vi "PRY_to_Quat.vi"(1 "From Degrees? (T)":bool=TRUE, 2 "Orientation":T1) -> (0 "Quaternion":cluster{"x":dbl, "y":dbl, "z":dbl, "w":dbl})   [LabVIEW 2014]
doc: "Converts a Pitch, Roll, Yaw orientation to a Quaternion"
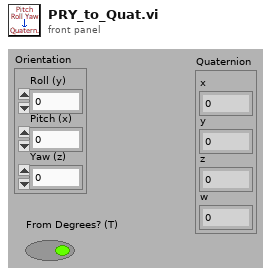
[diagram p1: front panel]
types:
  T1 = cluster{"Roll (y)":dbl, "Pitch (x)":dbl, "Yaw (z)":dbl}
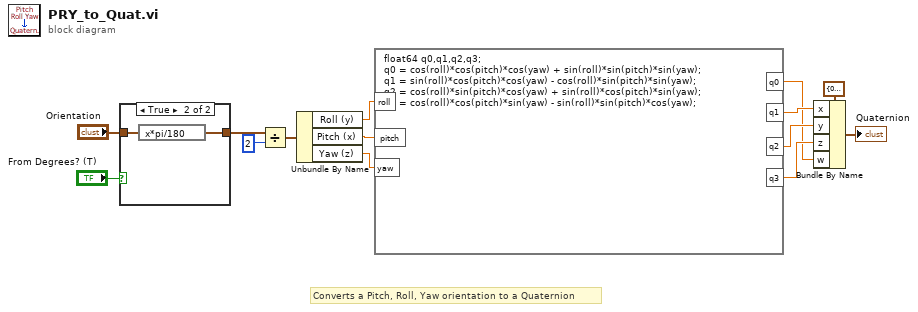
[diagram p0: block diagram]
diagram:
  # "Converts a Pitch, Roll, Yaw orientation to a Quaternion"
  n1 = case shown="True" "From Degrees? (T)" {
    tunnel: "Orientation" -> [w15 w17]
    tunnel: [w15 w16] -> w1
    frame False {
    }
    frame True {
      n2 = expression code="x*pi/180"(w17) -> (w16:T1)
    }
  }
  n3 = Divide(x=w1, y=2) -> (x/y=w14:T1)
  n4 = Unbundle By Name(w14) -> ("Roll (y)"=w13:dbl, "Pitch (x)"=w12:dbl, "Yaw (z)"=w11:dbl)
  n5 = formula code="float64 q0,q1,q2,q3;\nq0 = cos(roll)*cos(pitch)*cos(yaw) + sin(roll)*sin(pitch)*sin(yaw);\nq1 = sin(roll)*cos(pitch)*cos(yaw) - cos(roll)*sin(pitch)*sin(yaw);\nq2 = cos(roll)*sin(pitch)*cos(yaw) + sin(roll)*cos(pitch)*sin(yaw);\nq3 = cos(roll)*cos(pitch)*sin(yaw) - sin(roll)*sin(pitch)*cos(yaw);"("roll"=w13, "pitch"=w12, "yaw"=w11) -> ("q0"=w6:dbl, "q1"=w9:dbl, "q2"=w8:dbl, "q3"=w7:dbl)
  n6 = Bundle By Name(cluster=cluster{"x":dbl, "y":dbl, "z":dbl, "w":dbl} {"x"=0.0, "y"=0.0, "z"=0.0, "w"=0.0} ("Orientation"), "x"=w9, "y"=w8, "z"=w7, "w"=w6) -> (→"Quaternion":cluster{"x":dbl, "y":dbl, "z":dbl, "w":dbl})
